vi "Write_INI_File.vi"(8 "Status/Errors in":refnum<vi>, 9 "Control Parameters [] in":T1[](array[typedef]) {"Aux Byte Value" format="%02x"; "Max Real Value" format="%#_6e"; "Min Real Value" format="%#_6e"; "dReal/dByte" format="%#_6e"; "Byte Value" format="%02x"; "Identifier" format="%02x"}, 10 "Path configuration file in":path, 11 "Path ini file in":path) -> (0 "Status/Errors out":refnum<vi>, 1 "Error?":bool, 2 "Path configuration file out":path, 3 "Path ini file out":path)   [LabVIEW 2010]
uses:
  Controls/Control_Parameters.ctl
  Controls/Master.ctl
  Controls/Configuration_File_Parameters.ctl
  Controls/Mode.ctl
  Controls/Configuration_File_Elements.ctl
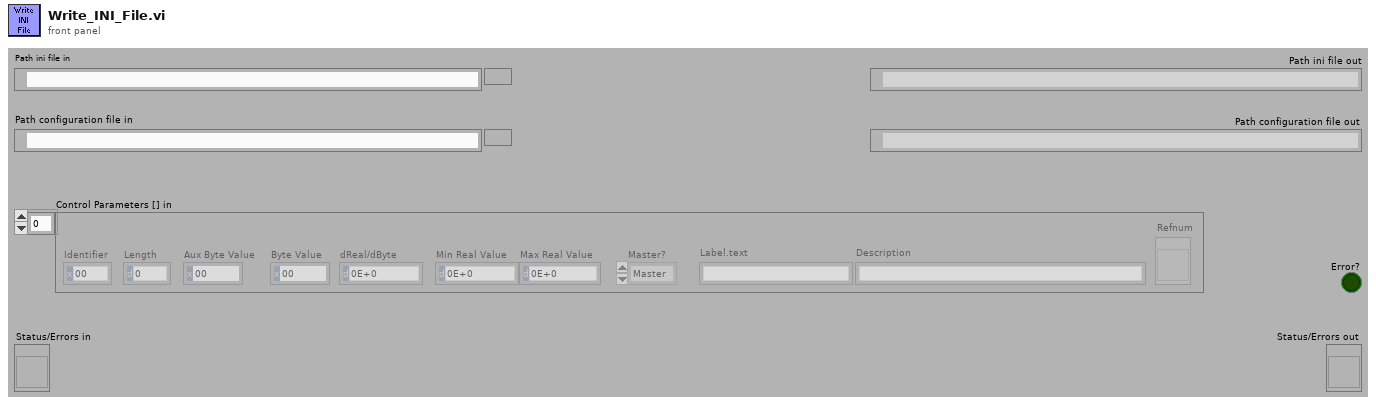
[diagram p1: front panel]
types:
  T1 = typedef "Control_Parameters.ctl" = cluster{"Identifier":u8, "Length":u16, "Byte Value":u32, "dReal/dByte":dbl, "Min Real Value":dbl, "Max Real Value":dbl, "Master?":T2, "Label.text":string, "Description":string, "Refnum":refnum<vi>, "Aux Byte Value":u32}
  T2 = typedef "Master.ctl" = enum16{"Master", "Slave", "General"}
  T3 = enum16{"open", "open or create", "create or replace", "create", "open (read only)"}
  T4 = typedef "Configuration_File_Parameters.ctl" = cluster{"Mode":T5, "Hardware":enum8{"None", "HiSPARC I", "HiSPARC II", "HiSPARC III"}, "Time difference":string}
  T5 = typedef "Mode.ctl" = cluster{"Mode":enum8{"Stop", "Dialog", "Hisparc II", "Hisparc II DAQ", "Alignment"}, "Expert?":bool, "Dialog?":bool}
  T6 = typedef "Configuration_File_Elements.ctl" = enum16{"None", "All", "Mode", "Hardware", "Time difference"}
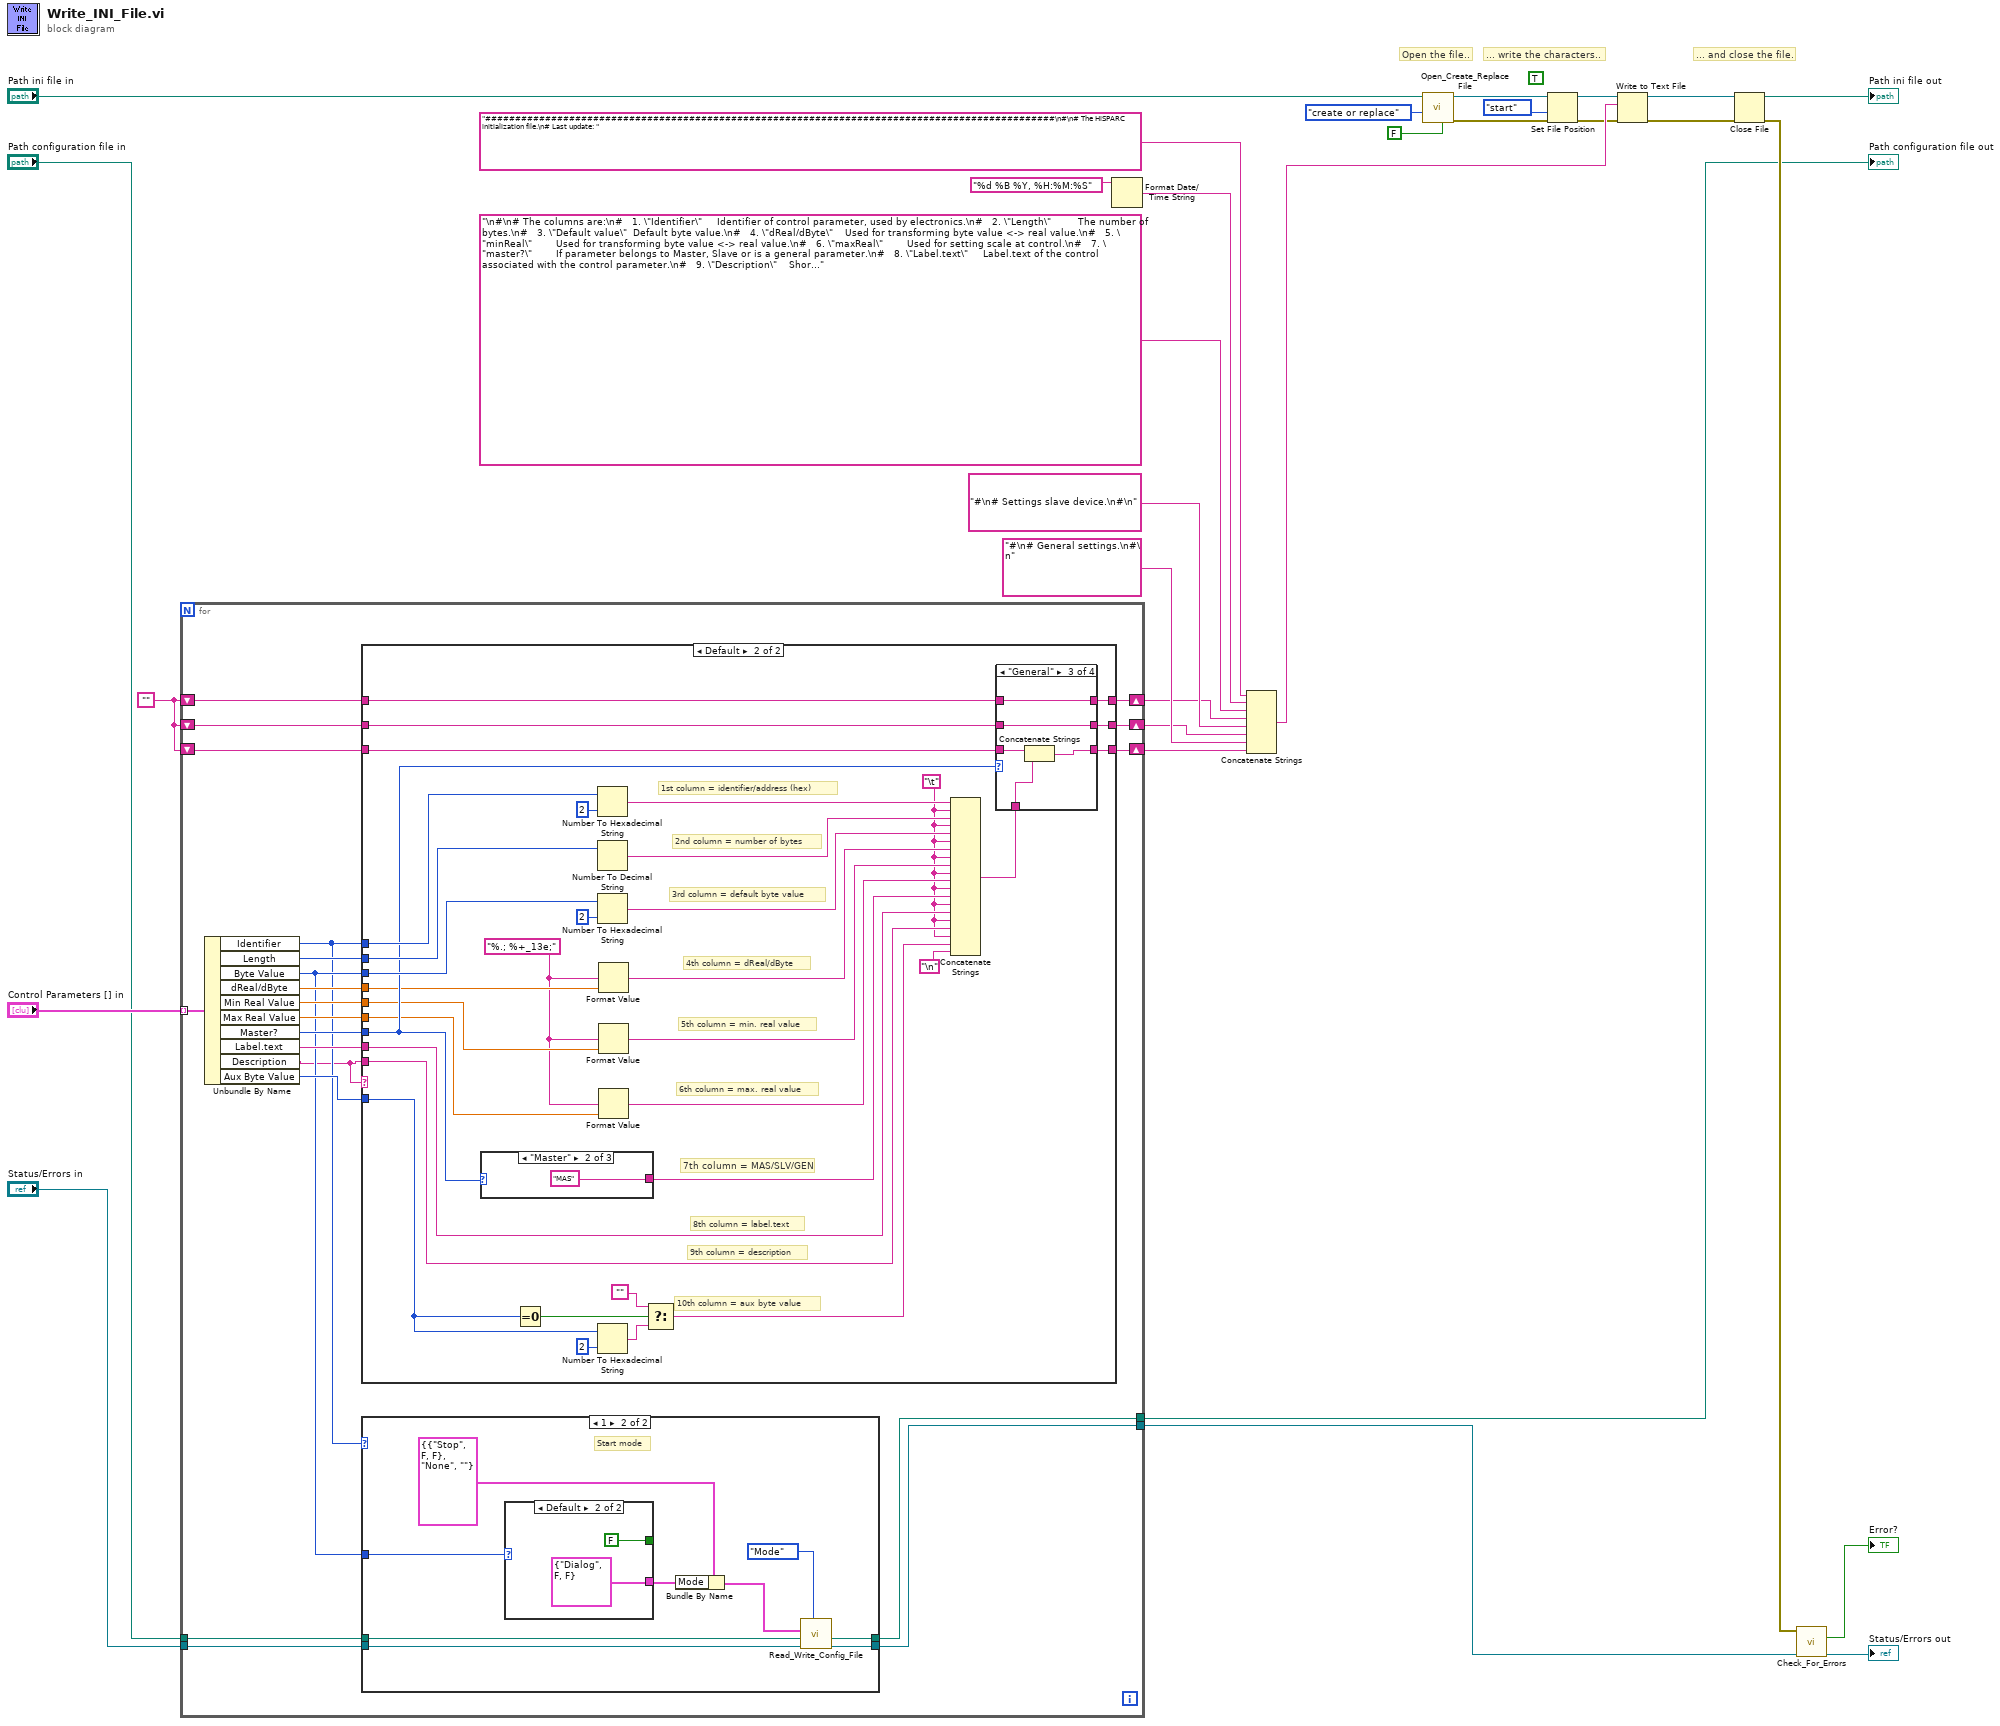
[diagram p0: block diagram]
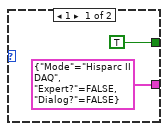
[diagram p3: hidden frame]
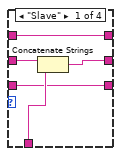
[diagram p5: hidden frame]
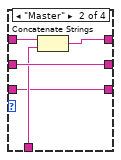
[diagram p6: hidden frame]
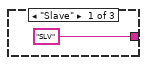
[diagram p8: hidden frame]
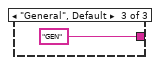
[diagram p9: hidden frame]
diagram:
  (unwired) TRUE
  w25 = ""
  # "... and close the file."
  # "... write the characters.."
  # "Open the file.."
  n1 = for {
    tunnel: "Control Parameters [] in" -> [w51] mode=indexing
    shift-right: [w43] -> w20
    shift-left: w25 -> [w50]
    shift-right: [w42] -> w21
    shift-left: w25 -> [w40]
    shift-right: [w41] -> w22
    shift-left: w25 -> [w39]
    tunnel: "Path configuration file in" -> [w35]
    tunnel: "Status/Errors in" -> [w37]
    tunnel: [w36] -> w6
    tunnel: [w34] -> w5
    n2 = Unbundle By Name(w51) -> ("Identifier"=w32:u8, "Length"=w49:u16, "Byte Value"=w33:u32, "dReal/dByte"=w48:dbl, "Min Real Value"=w47:dbl, "Max Real Value"=w46:dbl, "Master?"=w45:T2, "Label.text"=w44:string, "Description"=w31:string, "Aux Byte Value"=w38:u32)
    n3 = case shown="Default" w31 {
      tunnel: w50 -> [w69 w87]
      tunnel: w32 -> [_ w103]
      tunnel: w49 -> [_ w97]
      tunnel: w33 -> [_ w96]
      tunnel: w48 -> [_ w79]
      tunnel: w47 -> [_ w78]
      tunnel: w46 -> [_ w80]
      tunnel: w45 -> [_ w88]
      tunnel: w44 -> [_ w92]
      tunnel: w31 -> [_ w90]
      tunnel: [w69 w85] -> w43
      tunnel: [w68 w84] -> w42
      tunnel: [w67 w83] -> w41
      tunnel: w40 -> [w68 w82]
      tunnel: w39 -> [w67 w81]
      tunnel: w38 -> [_ w72]
      frame "" {
        # "If there is no description, then the control parameter does not belong in the file.\n(This is the case for parameters associated with e.g. the traces, the statistics, etc.)"
      }
      frame Default {
        w77 = "%.; %+_13e;"
        w76 = "\t"
        # "10th column = aux byte value"
        # "6th column = max. real value"
        # "9th column = description"
        # "8th column = label.text"
        # "7th column = MAS/SLV/GEN"
        # "5th column = min. real value"
        # "4th column = dReal/dByte"
        # "3rd column = default byte value"
        # "2nd column = number of bytes"
        # "1st column = identifier/address (hex)"
        n4 = case shown="\"Master\"" w88 {
          tunnel: ["SLV" "MAS" "GEN"] -> w91
          frame "Slave" {
          }
          frame "Master" {
          }
          frame "General", Default {
          }
        }
        n5 = Equal To 0?(x=w72) -> (x = 0?=w71:bool)
        n6 = Number To Hexadecimal String(1:i16 2 ("width (-)"), 2:w103) -> (0:w101:string)
        n7 = Number To Decimal String(number=w97) -> (decimal integer string=w99:string)  [unwired: 1 out]
        n8 = Number To Hexadecimal String(1:i16 2 ("width (-)"), 2:w96) -> (0:w98:string)
        n9 = Number To Hexadecimal String(1:i16 2 ("width (-)"), 2:w72) -> (0:w74:string)
        n10 = Format Value(format string=w77, value (0)=w79) -> (output string=w95:string)  [unwired: 1 in]
        n11 = Format Value(format string=w77, value (0)=w78) -> (output string=w94:string)  [unwired: 1 in]
        n12 = Format Value(format string=w77, value (0)=w80) -> (output string=w93:string)  [unwired: 1 in]
        n13 = Select(t="", s=w71, f=w74) -> (s? t:f=w70:string)
        n14 = Concatenate Strings(w101, w76, w99, w76, w98, w76, w95, w76, w94, w76, w93, w76, w91, w76, w92, w76, w90, w76, w70, "\n") -> (w86:string)
        n15 = case shown="\"General\"" w88 {
          tunnel: w87 -> [w104 w109 w118 w121]
          tunnel: w86 -> [w106 w110 w117 _]
          tunnel: [w104 w109 w116 w121] -> w85
          tunnel: [w105 w111 w115 w120] -> w84
          tunnel: [w108 w112 w114 w119] -> w83
          tunnel: w82 -> [w107 w111 w115 w120]
          tunnel: w81 -> [w108 w113 w114 w119]
          frame "Slave" {
            n16 = Concatenate Strings(w107, w106) -> (w105:string)
          }
          frame "Master" {
            n17 = Concatenate Strings(w113, w110) -> (w112:string)
          }
          frame "General" {
            n18 = Concatenate Strings(w118, w117) -> (w116:string)
          }
          frame Default {
          }
        }
      }
    }
    n19 = case shown="1" w32 {
      tunnel: w37 -> [w52 w58]
      tunnel: [w52 w57] -> w36
      tunnel: w35 -> [w53 w56]
      tunnel: [w53 w55] -> w34
      tunnel: w33 -> [_ w54]
      frame Default {
      }
      frame 1 {
        # "Start mode"
        n20 = case shown="Default" w54 {
          tunnel: [TRUE FALSE] -> _
          tunnel: [T5 {"Mode"=enum."Hisparc II DAQ", "Expert?"=FALSE, "Dialog?"=FALSE} ("Mode in") T5 {"Mode"=enum."Dialog", "Expert?"=FALSE, "Dialog?"=FALSE} ("Mode in")] -> w61
          frame 1 {
          }
          frame Default {
          }
        }
        n21 = Bundle By Name(cluster=T4 {"Mode"={"Mode"=enum."Stop", "Expert?"=FALSE, "Dialog?"=FALSE}, "Hardware"=enum."None", "Time difference"=""} ("Parameters in"), "Mode"=w61) -> (w62:T4)
        n22 = call "Read_Write_Config_File.vi"("Element (None)"=Configuration_File_Elements."Mode", "Status/Errors in"=w58, "Path config file in"=w56, "Parameters in"=w62) -> ("Status/Errors out"=w57:refnum<vi>, "Path config file out"=w55:path)  [unwired: 1 in, 5 out]
      }
    }
  }
  "Path configuration file out" <- w5
  n23 = Format Date/Time String(time format string (%c)="%d %B %Y, %H:%M:%S") -> (date/time string=w28:string)  [unwired: 2 out]
  n24 = Concatenate Strings("###############################################################################################\n#\n# The HiSPARC initialization file.\n# Last update: ", w28, "\n#\n# The columns are:\n#   1. \"Identifier\"     Identifier of control parameter, used by electronics.\n#   2. \"Length\"         The number of bytes.\n#   3. \"Default value\"  Default byte value.\n#   4. \"dReal/dByte\"    Used for transforming byte value <-> real value.\n#   5. \"minReal\"        Used for transforming byte value <-> real value.\n#   6. \"maxReal\"        Used for setting scale at control.\n#   7. \"master?\"        If parameter belongs to Master, Slave or is a general parameter.\n#   8. \"Label.text\"     Label.text of the control associated with the control parameter.\n#   9. \"Description\"    Short description of the control parameter.\n#\n###############################################################################################\n#\n# Settings master device.\n#\n", w22, "#\n# Settings slave device.\n#\n", w21, "#\n# General settings.\n#\n", w20) -> (w10:string)
  n25 = call <vilib>:"Open_Create_Replace File.vi"("advisory dialog? (display:T)"=FALSE, "function (open:0)"=T3."create or replace", "file path"="Path ini file in") -> ("error out"=w9:errorcluster, "refnum"=w16:refnum<file>)  [unwired: 4 in, 3 out]
  n26 = Set File Position(refnum=w16, from (0:start)=enum16{"start", "end", "current"}."start" ("pos mode (0:2)"), error in=w9) -> (refnum out=w3:refnum<file>, error out=w2:errorcluster)  [unwired: 1 out]
  n27 = Write to Text File(file (use dialog)=w3, text=w10, error in=w2) -> (refnum out=w12:refnum<file>, error out=w8:errorcluster)  [unwired: 2 out]
  n28 = Close File(refnum=w12, error in=w8) -> (path=→"Path ini file out":path, error out=w13:errorcluster)
  n29 = call "Check_For_Errors.vi"("Status/Errors in"=w6, "error in"=w13) -> ("Status/Errors out"=→"Status/Errors out":refnum<vi>, "Status"=→"Error?":bool)  [unwired: 8 out]
